vi "ma_SML Averaged FFT Spectrum.vi"(6 "reset averagering?":bool, 8 "error in (no error)":errorcluster, 9 "averaging parameters":T1={"averaging type"=enum."no averaging", "averaging settings"={"weighting type"=enum."linear", "weighting settings"={"size"=10.0, "linear weighting mode"=enum."moving average"}}}, 10 "spectral info in":T3 {"window" items=["Rectangle"=0, "Hanning"=1, "Hamming"=2, "Blackman-Harris"=3, "Exact Blackman"=4, "Blackman"=5, "Flat Top"=6, "4 Term B-Harris "=7, "7 Term B-Harris"=8, "Low Sidelobe"=9, "Blackman Nuttall"=11, "Triangle"=30, "Bartlett-Hanning"=31, "Bohman"=32, "Parzen"=33, "Welch"=34, "Kaiser"=60, "Dolph-Chebyshev"=61, "Gaussian"=62]}, 11 "FFT Spectrum":T4 {"spectrum" format="%.2f"; "df" format="%.2f"; "f0" format="%.2f"}) -> (0 "error out":errorcluster, 1 "data ready?":bool, 2 "spectral info out":T3 {"window" items=["Rectangle"=0, "Hanning"=1, "Hamming"=2, "Blackman-Harris"=3, "Exact Blackman"=4, "Blackman"=5, "Flat Top"=6, "4 Term B-Harris "=7, "7 Term B-Harris"=8, "Low Sidelobe"=9, "Blackman Nuttall"=11, "Triangle"=30, "Bartlett-Hanning"=31, "Bohman"=32, "Parzen"=33, "Welch"=34, "Kaiser"=60, "Dolph-Chebyshev"=61, "Gaussian"=62]}, 3 "avg FFT spectrum":T4 {"spectrum" format="%.2f"; "df" format="%.2f"; "f0" format="%.2f"}, 4 "averages sofar":dbl)   [LabVIEW 2020, in "NI_MAPro.lvlib"]
uses:
  NI_MAPro.lvlib
  ma_sml_Spectrum Cluster (complex).ctl
  ma_sml_Spectral Info.ctl
  ma_sml_Averaging Parameters.ctl
  ma_sml_Averaging Settings.ctl
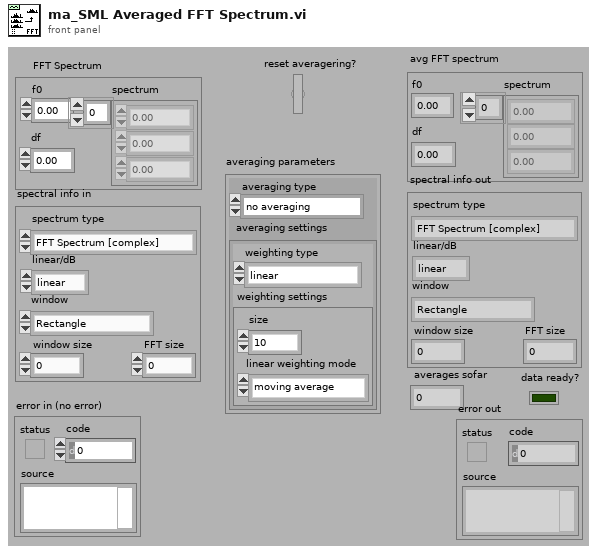
[diagram p1: front panel]
types:
  T1 = typedef "NI_MAPro.lvlib/ma_sml_Averaging Parameters.ctl" = cluster{"averaging type":enum16{"no averaging", "vector averaging", "RMS averaging", "peak hold"}, "averaging settings":T2}
  T2 = typedef "NI_MAPro.lvlib/ma_sml_Averaging Settings.ctl" = cluster{"weighting type":enum16{"linear", "exponential"}, "weighting settings":cluster{"size":dbl, "linear weighting mode":enum16{"one shot", "auto restart one shot", "moving average", "continuous"}}}
  T3 = typedef "NI_MAPro.lvlib/ma_sml_Spectral Info.ctl" = cluster{"spectrum type":enum16{"FFT Spectrum [complex]", "Amplitude [Magnitude]", "Power [Magnitude^2]", "Cross Spectrum [complex]", "Frequency Response [Complex]"}, "linear/dB":enum16{"linear", "dB"}, "window":u16, "window size":i32, "FFT size":i32}
  T4 = typedef "NI_MAPro.lvlib/ma_sml_Spectrum Cluster (complex).ctl" = cluster{"f0":dbl, "df":dbl, "spectrum":cdb[]}
  T5 = enum16{"no averaging", "vector averaging", "RMS averaging", "peak hold"}
  T6 = enum16{"FFT Spectrum [complex]", "Amplitude [Magnitude]", "Power [Magnitude^2]", "Cross Spectrum [complex]", "Frequency Response [Complex]"}
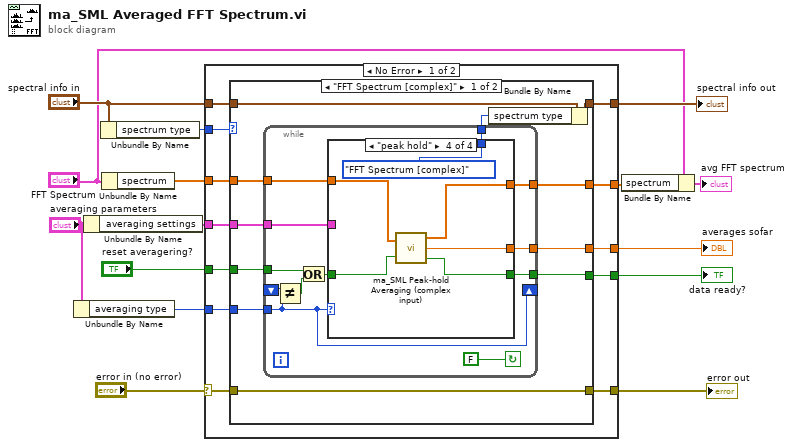
[diagram p0: block diagram]
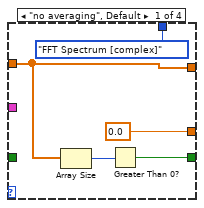
[diagram p2: hidden frame]
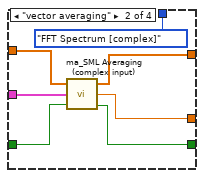
[diagram p3: hidden frame]
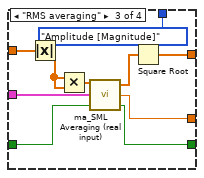
[diagram p4: hidden frame]
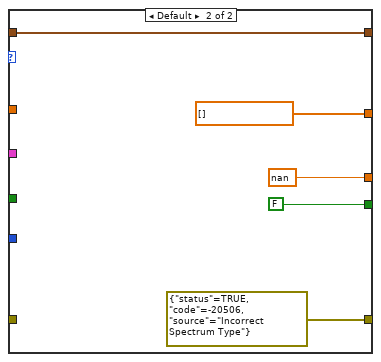
[diagram p5: hidden frame]
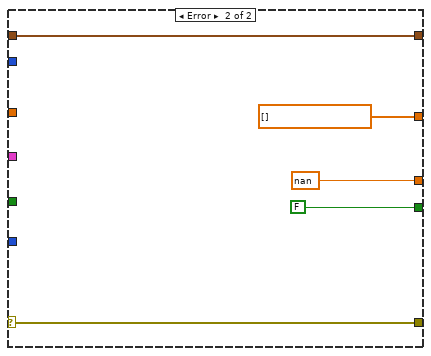
[diagram p6: hidden frame]
diagram:
  n1 = Unbundle By Name("averaging parameters") -> ("averaging type"=w5:T5)
  n2 = Unbundle By Name("averaging parameters") -> ("averaging settings"=w6:T2)
  n3 = Unbundle By Name("spectral info in") -> ("spectrum type"=w12:T6)
  n4 = Unbundle By Name("FFT Spectrum") -> ("spectrum"=w13:cdb[])
  n5 = case shown="No Error" "error in (no error)" {
    selector: "error in (no error)" -> [w16 w84]
    tunnel: w13 -> [w22 _]
    tunnel: [w27 cdb[] [] ("y")] -> w7
    tunnel: [w21 FALSE] -> w14
    tunnel: [w26 nan ("Averaged So-far")] -> w15
    tunnel: "reset averagering?" -> [w25 _]
    tunnel: w5 -> [w24 _]
    tunnel: w6 -> [w23 _]
    tunnel: w12 -> [w20 _]
    tunnel: [w19 w84] -> w3
    tunnel: "spectral info in" -> [w18 w85]
    tunnel: [w17 w85] -> w10
    frame No Error {
      n6 = case shown="\"FFT Spectrum [complex]\"" w20 {
        tunnel: [w38 cdb[] []] -> w27
        tunnel: [w37 nan ("Averaged So-far")] -> w26
        tunnel: w25 -> [w36 _]
        tunnel: w24 -> [w35 _]
        tunnel: w23 -> [w34 _]
        tunnel: w22 -> [w28 _]
        tunnel: [w29 FALSE] -> w21
        tunnel: w16 -> [w33 _]
        tunnel: [w33 errorcluster {"status"=TRUE, "code"=-20506, "source"="Incorrect Spectrum Type"} ("error in (no error)")] -> w19
        tunnel: w18 -> [w32 w79]
        tunnel: [w30 w79] -> w17
        frame "FFT Spectrum [complex]" {
          n7 = while {
            tunnel: [w41] -> w31
            tunnel: w34 -> [w43]
            shift-left: _ -> [w45]
            shift-right: [w44] -> _
            tunnel: w35 -> [w44]
            tunnel: w36 -> [w40]
            tunnel: [w47] -> w37
            tunnel: [w48] -> w29
            tunnel: [w49] -> w38
            tunnel: w28 -> [w50]
            stop <- FALSE continue-if-true
            n8 = Not Equal?(x=w45, y=w44) -> (x != y?=w39:bool)
            n9 = Or(x=w40, y=w39) -> (x .or. y?=w46:bool)
            n10 = case shown="\"peak hold\"" w44 {
              tunnel: [w54 w57 w68 w77] -> w49
              tunnel: w50 -> [w54 w62 w72 w75]
              tunnel: [w52 w59 w66 w74] -> w48
              tunnel: [0.0 ("Averaged So-far") w60 w67 w76] -> w47
              tunnel: w46 -> [_ w61 w65 w78]
              tunnel: w43 -> [_ w58 w64 _]
              tunnel: [T6."FFT Spectrum [complex]" ("spectrum type") T6."FFT Spectrum [complex]" ("spectrum type") T6."Amplitude [Magnitude]" ("spectrum type") T6."FFT Spectrum [complex]" ("spectrum type")] -> w41
              frame "no averaging", Default {
                n11 = Array Size(array=w54) -> (size(s)=w53:i32)
                n12 = Greater Than 0?(x=w53) -> (x > 0?=w52:bool)
              }
              frame "vector averaging" {
                n13 = call "ma_SML Averaging (complex input).vi"("reset?"=w61, "averaging settings"=w58, "x"=w62) -> ("data ready?"=w59:bool, "averaged sofar"=w60:dbl, "y"=w57:cdb[])
              }
              frame "RMS averaging" {
                n14 = Absolute Value(x=w72) -> (abs(x)=w70:dbl[])
                n15 = Multiply(x=w70, y=w70) -> (x*y=w71:dbl[])
                n16 = call "ma_SML Averaging (real input).vi"("reset?"=w65, "averaging settings"=w64, "x"=w71) -> ("data ready?"=w66:bool, "averaged sofar"=w67:dbl, "y"=w69:dbl[])
                n17 = Square Root(x=w69) -> (sqrt(x)=w68:dbl[])
              }
              frame "peak hold" {
                n18 = call "ma_SML Peak-hold Averaging (complex input).vi"("x"=w75, "reset?"=w78) -> ("y"=w77:cdb[], "averages sofar"=w76:dbl, "data ready?"=w74:bool)
              }
            }
          }
          n19 = Bundle By Name(cluster=w32, "spectrum type"=w31) -> (w30:T3)
        }
        frame Default {
        }
      }
    }
    frame Error {
    }
  }
  "averages sofar" <- w15
  "data ready?" <- w14
  "error out" <- w3
  "spectral info out" <- w10
  n20 = Bundle By Name(cluster="FFT Spectrum", "spectrum"=w7) -> (→"avg FFT spectrum":T4)
